vi "Image-GFV.vi"(8 "error in (no error)":errorcluster, 9 "Variant Input":variant, 10 "Input Image":T1, 11 "Image GFV Enum":T2=enum."Write") -> (0 "error out":errorcluster, 2 "Variant Output":variant, 3 "Output Image":T1)   [LabVIEW 2013]
doc: "Use this template to build a VI to use as a subVI."
uses:
  ImageEnum4GFV.ctl
  <vilib>/vision/Image Controls.llb/IMAQ Image.ctl
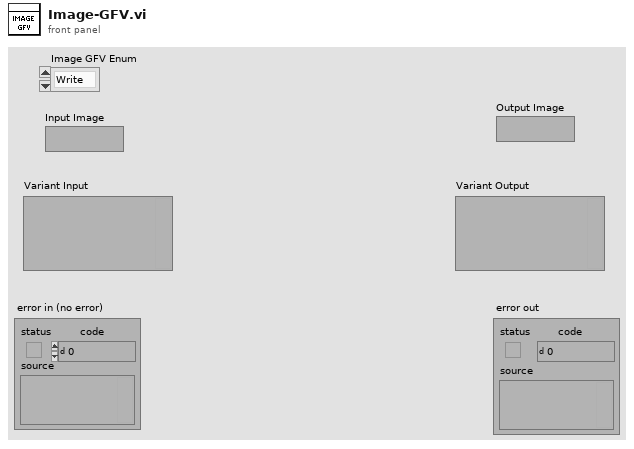
[diagram p1: front panel]
types:
  T1 = typedef "IMAQ Image.ctl" = refnum<image>
  T2 = typedef "ImageEnum4GFV.ctl" = enum16{"Delete", "Write", "Read", "Init"}
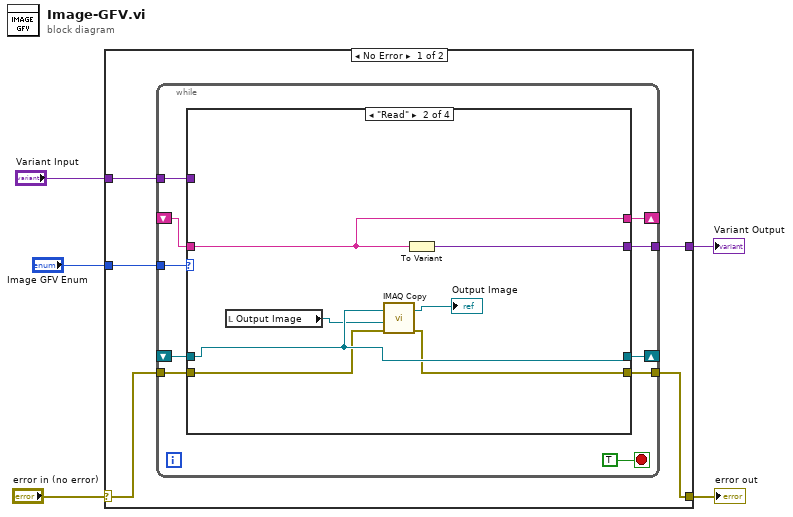
[diagram p0: block diagram]
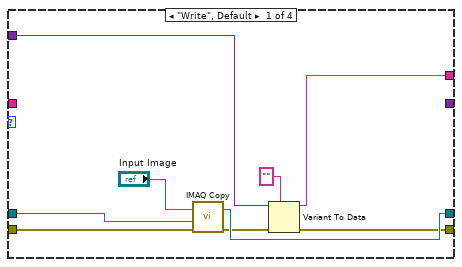
[diagram p2: hidden frame]
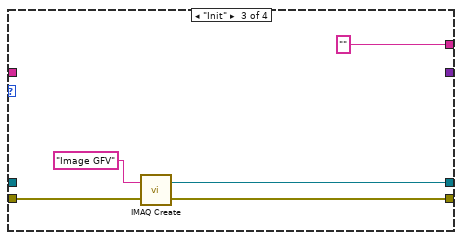
[diagram p3: hidden frame]
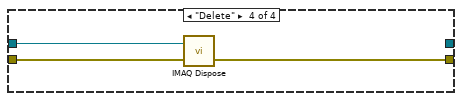
[diagram p4: hidden frame]
diagram:
  n1 = case shown="No Error" "error in (no error)" {
    selector: "error in (no error)" -> [w9 w45]
    tunnel: [w8 w45] -> w4
    tunnel: "Image GFV Enum" -> [w10 _]
    tunnel: "Variant Input" -> [w7 _]
    tunnel: [w6 _] -> w1
    frame No Error {
      n2 = while {
        tunnel: w10 -> [w19]
        tunnel: w9 -> [w18]
        tunnel: [w17] -> w8
        shift-right: [w16] -> _
        shift-left: _ -> [w15]
        shift-right: [w14] -> _
        shift-left: _ -> [w12]
        tunnel: w7 -> [w13]
        tunnel: [w11] -> w6
        stop <- TRUE stop-if-true
        n3 = case shown="\"Read\"" w19 {
          tunnel: w18 -> [w27 w33 w40 w44]
          tunnel: [w22 w32 w39 w43] -> w17
          tunnel: [w28 w36 w38 _] -> w16
          tunnel: w15 -> [w29 w36 _ w42]
          tunnel: [w21 w30 "" ("Image Name") _] -> w14
          tunnel: w13 -> [w25 _ _ _]
          tunnel: w12 -> [_ w30 _ _]
          tunnel: [_ w31 _ _] -> w11
          frame "Write", Default {
            n4 = call "IMAQ Copy"("error in (no error)"=w27, "Image Dst"=w29, "Image Src"="Input Image") -> ("error out"=w23:errorcluster, "Image Dst Out"=w28:T1)  [unwired: 3 in]
            n5 = Variant To Data(error in=w23, type="" ("Image Name"), Variant=w25) -> (data=w21:string, error out=w22:errorcluster)
          }
          frame "Read" {
            n6 = local read "Output Image"() -> (w35:T1)
            n7 = call "IMAQ Copy"("error in (no error)"=w33, "Image Dst"=w35, "Image Src"=w36) -> ("error out"=w32:errorcluster, "Image Dst Out"=→"Output Image":T1)  [unwired: 3 in]
            n8 = To Variant(anything=w30) -> (Variant=w31:variant)
          }
          frame "Init" {
            n9 = call "IMAQ Create"("Image Name"="Image GFV", "error in (no error)"=w40) -> ("New Image"=w38:T1, "error out"=w39:errorcluster)  [unwired: 2 in, 1 out]
          }
          frame "Delete" {
            n10 = call "IMAQ Dispose"("Image"=w42, "error in (no error)"=w44) -> ("error out"=w43:errorcluster)  [unwired: 1 in, 3 out]
          }
        }
      }
    }
    frame Error {
    }
  }
  "error out" <- w4
  "Variant Output" <- w1
